vi "Left-Right ring to Text.vi"(1 "Ear":T1=enum."Left") -> (0 "Left/Right":string)   [LabVIEW 2020]
uses:
  Left-Right ring.ctl
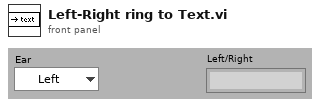
[diagram p1: front panel]
types:
  T1 = typedef "Left-Right ring.ctl" = enum16{"Right", "Left"}
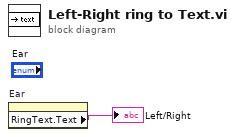
[diagram p0: block diagram]
diagram:
  n1 = property on="Ear" class="Enum (strict)"() -> ("RingText.Text"=→"Left/Right":string)  [unwired: 2 in, 2 out]
